vi "Benchmark mupLib_eval_bulk.vi"(8 "error in (no error)":errorcluster, 10 "Iterations":i32, 11 "Expression":string) -> (0 "error out":errorcluster, 2 "x":dbl[](array[numeric]), 3 "y":dbl[](array[numeric]), 5 "dt average":dbl)   [LabVIEW 2015]
uses:
  mupLib/mupLibPath.vi
  mupLib/mupCheckError.vi
  <vilib>/Utility/error.llb/Error Cluster From Error Code.vi
  mupLib/mupLib.lvlib
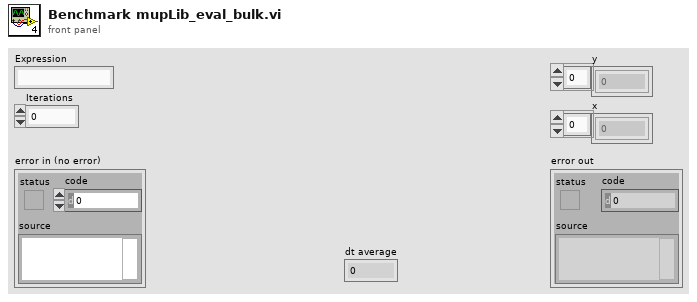
[diagram p1: front panel]
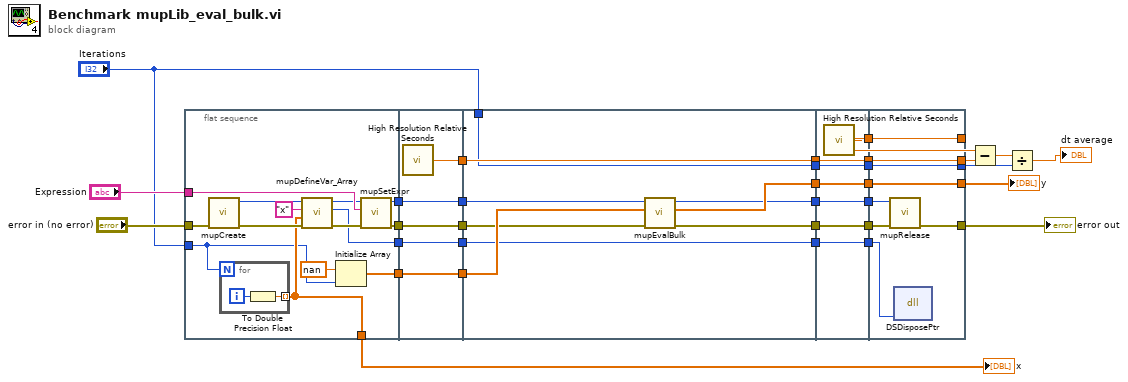
[diagram p0: block diagram]
diagram:
  n1 = flat-sequence {
    tunnel: [w44] -> w18
    tunnel: "Expression" -> [w46]
    tunnel: "error in (no error)" -> [w47]
    tunnel: [w45] -> w16
    tunnel: [w38] -> w14
    tunnel: "Iterations" -> [w36]
    tunnel: [w37] -> w3
    tunnel: [w34] -> w1
    tunnel: [w54] -> w32
    tunnel: [w53] -> w28
    tunnel: w18 -> [w54]
    tunnel: [w52] -> w17
    tunnel: w16 -> [w52]
    tunnel: [w51] -> w15
    tunnel: w14 -> [w51]
    tunnel: [w50] -> w2
    tunnel: w1 -> [w50]
    tunnel: w32 -> [w56]
    tunnel: [w63] -> w31
    tunnel: [w62] -> w30
    tunnel: [w61] -> w29
    tunnel: w28 -> [w61]
    tunnel: "Iterations" -> [w60]
    tunnel: [w60] -> w23
    tunnel: w17 -> [w59]
    tunnel: w15 -> [w55]
    tunnel: [w58] -> w7
    tunnel: [w55] -> w5
    tunnel: w2 -> [w57]
    tunnel: w31 -> [w70]
    tunnel: w30 -> [w69]
    tunnel: w29 -> [w68]
    tunnel: w23 -> [w66]
    tunnel: [w70] -> w13
    tunnel: [w69] -> w12
    tunnel: [w68] -> w11
    tunnel: [w67] -> w10
    tunnel: [w66] -> w9
    tunnel: [w65] -> w8
    tunnel: w7 -> [w65]
    tunnel: [w64] -> w6
    tunnel: w5 -> [w64]
    tunnel: [w75] -> w24
    tunnel: [w76] -> w27
    tunnel: [w77] -> w26
    tunnel: [w78] -> w33
    tunnel: [w73] -> w19
    tunnel: w13 -> [w74]
    tunnel: w12 -> [w78]
    tunnel: w11 -> [w77]
    tunnel: w10 -> [w76]
    tunnel: w9 -> [w75]
    tunnel: w8 -> [w72]
    tunnel: w6 -> [w71]
    frame #0 {
      n2 = call "mupCreate.vi"("error in (no error)"=w47) -> ("error out"=w42:errorcluster, "hParser out"=w43:u64)  [unwired: 9 in]
      n3 = for {
        N: w36 -> [_]
        tunnel: [w48] -> w37 mode=indexing
        i -> [w49]
        n4 = To Double Precision Float(number=w49) -> (double precision float=w48:dbl)
      }
      n5 = call "mupDefineVar_Array.vi"("error in (no error)"=w42, "initValue"=w37, "varName"="x", "hParser in"=w43) -> ("error out"=w40:errorcluster, "varAddr"=w38:u64, "hParser out"=w39:u64)  [unwired: 5 in]
      n6 = Initialize Array(nan ("element"), w36) -> (w34:dbl[])
      n7 = call "mupSetExpr.vi"("error in (no error)"=w40, "szExpr"=w46, "muPar in"=w39) -> ("error out"=w44:errorcluster, "muPar out"=w45:u64)  [unwired: 7 in]
    }
    frame #1 {
      n8 = call <vilib>:"High Resolution Relative Seconds.vi"() -> ("relative seconds"=w53:dbl)
    }
    frame #2 {
      n9 = call "mupEvalBulk.vi"("error in (no error)"=w56, "a_res"=w57, "hParser in"=w59) -> ("error out"=w63:errorcluster, "results"=w62:dbl[], "hParser out"=w58:u64)  [unwired: 6 in]
    }
    frame #3 {
      n10 = call <vilib>:"High Resolution Relative Seconds.vi"() -> ("relative seconds"=w67:dbl)
    }
    frame #4 {
      n11 = call "mupRelease.vi"("error in (no error)"=w74, "hParser in"=w72) -> ("error out"=w73:errorcluster)  [unwired: 9 in]
      n12 = dll-call lib="LabVIEW" fn="DSDisposePtr"("ptr"=w71) -> ()  [unwired: 5 in, 2 out]
    }
  }
  n13 = Subtract(x=w27, y=w26) -> (x-y=w25:dbl)
  n14 = Divide(x=w25, y=w24) -> (x/y=→"dt average":dbl)
  "y" <- w33
  "x" <- w3
  "error out" <- w19
